vi "Simple LED Example_09.vi"() -> ()   [LabVIEW 2016]
uses:
  <vilib>/LabVIEW Interface for Arduino/Type Defs/Pin Mode.ctl
  <vilib>/LabVIEW Interface for Arduino/LabVIEW Interface for Arduino.lvlib
panel:
  in  "Digital I/O Pin":u8
  in  "Value (0)":u8
  in  "Stop":bool
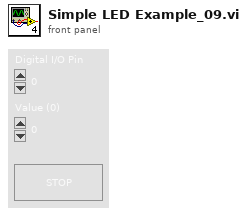
[diagram p1: front panel]
types:
  T1 = typedef "LabVIEW Interface for Arduino.lvlib/Pin Mode.ctl" = enum8{"Input", "Output"}
  T2 = typedef "LabVIEW Interface for Arduino.lvlib/Arduino Resource.ctl" = cluster{"VISA resource":refnum<visa-resource-name>, "Board Type":T3, "Connection Type":enum8{"USB / Serial"}, "Bytes Per Packet (15)":u8}
  T3 = typedef "LabVIEW Interface for Arduino.lvlib/Board Type.ctl" = enum16{"Uno", "Dimuelanove w/Atmega 328", "Mega 2560"}
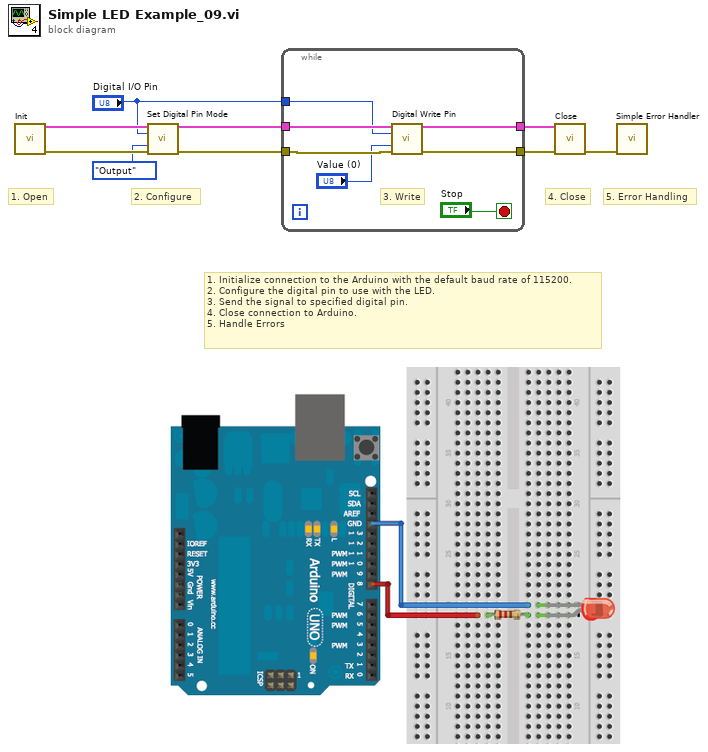
[diagram p0: block diagram]
diagram:
  # "5. Error Handling"
  # "4. Close"
  # "2. Configure"
  # "1. Open"
  # "1. Initialize connection to the Arduino with the default baud rate of 115200.\n2. Configure the digital pin to use with the LED.\n3. Send the signal to specified digital pin.\n4. Close connection to Arduino.\n5. Handle Errors"
  n1 = call <vilib>:"Init.vi"() -> ("Arduino Resource"=w6:T2, "error out"=w5:errorcluster)  [unwired: 18 in]
  n2 = call <vilib>:"Set Digital Pin Mode.vi"("Arduino Resource"=w6, "Digital I/O Pin"="Digital I/O Pin", "Pin Mode (Input)"=Pin_Mode."Output", "error in"=w5) -> ("Arduino Resource"=w4:T2, "error out"=w3:errorcluster)  [unwired: 10 in]
  n3 = while {
    tunnel: [w16] -> w8
    tunnel: w4 -> [w13]
    tunnel: w3 -> [w14]
    tunnel: [w15] -> w7
    tunnel: "Digital I/O Pin" -> [w11]
    stop <- "Stop" stop-if-true
    # "3. Write"
    n4 = call <vilib>:"Digital Write Pin.vi"("Arduino Resource"=w13, "Digital I/O Pin (0)"=w11, "Value (0)"="Value (0)", "error in"=w14) -> ("Arduino Resource"=w16:T2, "error out"=w15:errorcluster)  [unwired: 10 in]
  }
  n5 = call <vilib>:"Close.vi"("Arduino Resource"=w8, "error in"=w7) -> ("error out"=w9:errorcluster)  [unwired: 13 in]
  n6 = call <vilib>:"Simple Error Handler.vi"("error in (no error)"=w9) -> ()  [unwired: 4 in, 5 out]
